vi "Edit Auton Queue Order.vi"(10 "Boolean":bool, 11 "Manip Button":T1) -> ()   [LabVIEW 2015]
uses:
  Common Code/Gamepads/Button Cluster.ctl
  Common Code/Change Detect.vi
  Common Code/Change Detect Boolean.vi
  Robot Global Data.vi
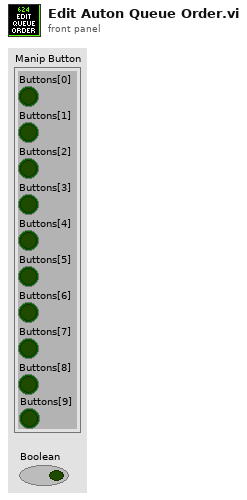
[diagram p1: front panel]
types:
  T1 = typedef "Button Cluster.ctl" = cluster{"Buttons[0]":bool, "Buttons[1]":bool, "Buttons[2]":bool, "Buttons[3]":bool, "Buttons[4]":bool, "Buttons[5]":bool, "Buttons[6]":bool, "Buttons[7]":bool, "Buttons[8]":bool, "Buttons[9]":bool}
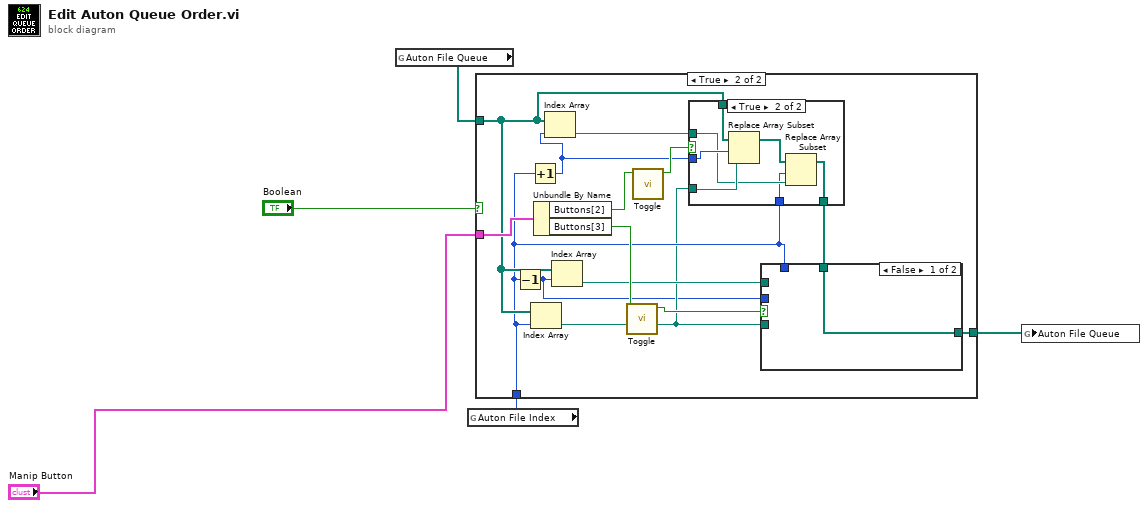
[diagram p0: block diagram]
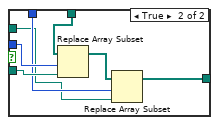
[diagram p3: hidden frame]
diagram:
  n1 = global read "Robot Global Data.vi" "Auton File Queue"() -> (w4:path[])
  n2 = global read "Robot Global Data.vi" "Auton File Index"() -> (w3:i32)
  n3 = case shown="True" "Boolean" {
    tunnel: "Manip Button" -> [_ w20]
    tunnel: w3 -> [_ w12]
    tunnel: w4 -> [w6 w16]
    tunnel: [w6 w7] -> w5
    frame False {
    }
    frame True {
      n4 = Decrement(x=w12) -> (x-1=w8:i32)
      n5 = Increment(x=w12) -> (x+1=w15:i32)
      n6 = Index Array(array=w16, index=w12) -> (element=w10:path)
      n7 = Unbundle By Name(w20) -> ("Buttons[2]"=w19:bool, "Buttons[3]"=w18:bool)
      n8 = Index Array(array=w16, index=w15) -> (element=w14:path)
      n9 = Index Array(array=w16, index=w8) -> (element=w11:path)
      n10 = call "Toggle.vi"("In"=w18) -> ("Toggled"=w13:bool)  [unwired: 10 in]
      n11 = call "Toggle.vi"("In"=w19) -> ("Toggled"=w17:bool)  [unwired: 10 in]
      n12 = case shown="True" w17 {
        tunnel: w16 -> [w29 w36]
        tunnel: w15 -> [_ w35]
        tunnel: w10 -> [_ w34]
        tunnel: w14 -> [_ w32]
        tunnel: w12 -> [_ w31]
        tunnel: [w29 w30] -> w9
        frame False {
        }
        frame True {
          n13 = Replace Array Subset(array=w36, new element=w34, index=w35) -> (w33:path[])
          n14 = Replace Array Subset(array=w33, new element=w32, index=w31) -> (w30:path[])
        }
      }
      n15 = case shown="False" w13 {
        tunnel: w12 -> [_ w24]
        tunnel: w11 -> [_ w23]
        tunnel: w10 -> [_ w27]
        tunnel: w9 -> [w21 w28]
        tunnel: w8 -> [_ w26]
        tunnel: [w21 w22] -> w7
        frame False {
        }
        frame True {
          n16 = Replace Array Subset(array=w28, new element=w27, index=w26) -> (w25:path[])
          n17 = Replace Array Subset(array=w25, new element=w23, index=w24) -> (w22:path[])
        }
      }
    }
  }
  n18 = global write "Robot Global Data.vi" "Auton File Queue"(w5) -> ()
